vi "Status Queue.vi"(5 "All Status":bool, 7 "Action":T1=enum."Enqueue", 8 "Error In":errorcluster, 11 "Status Message [In]":string="Status Message") -> (0 "Error Out":errorcluster, 3 "Status Message [Out]":string="Status Message")   [LabVIEW 2017]
uses:
  Controls/Queue Manager Actions.ctl
  Controls/QueueNames.ctl
  Controls/MessagePacket.ctl
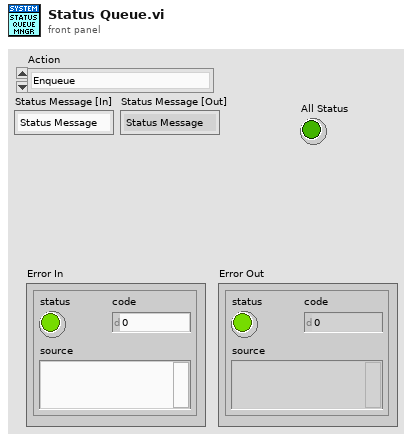
[diagram p1: front panel]
types:
  T1 = typedef "Queue Manager Actions.ctl" = enum16{"Init", "Enqueue", "Enqueue All", "Preview Queue", "Dequeue", "Get Status", "Flush Queue", "Flush All Queues", "Release All Queues", "Release Queue", "Enqueue at Opposite End"}
  T2 = typedef "MessagePacket.ctl" = cluster{"Message":string, "Parameter":variant}
  T3 = typedef "QueueNames.ctl" = enum16{"Main GUI", "Main Scan Processor", "Main Display", "Main Table Stage GUI", "Main Table Stage Proc.", "Scan Engine", "Vibratome GUI", "Vibratome Processor", "Slice Engine"}
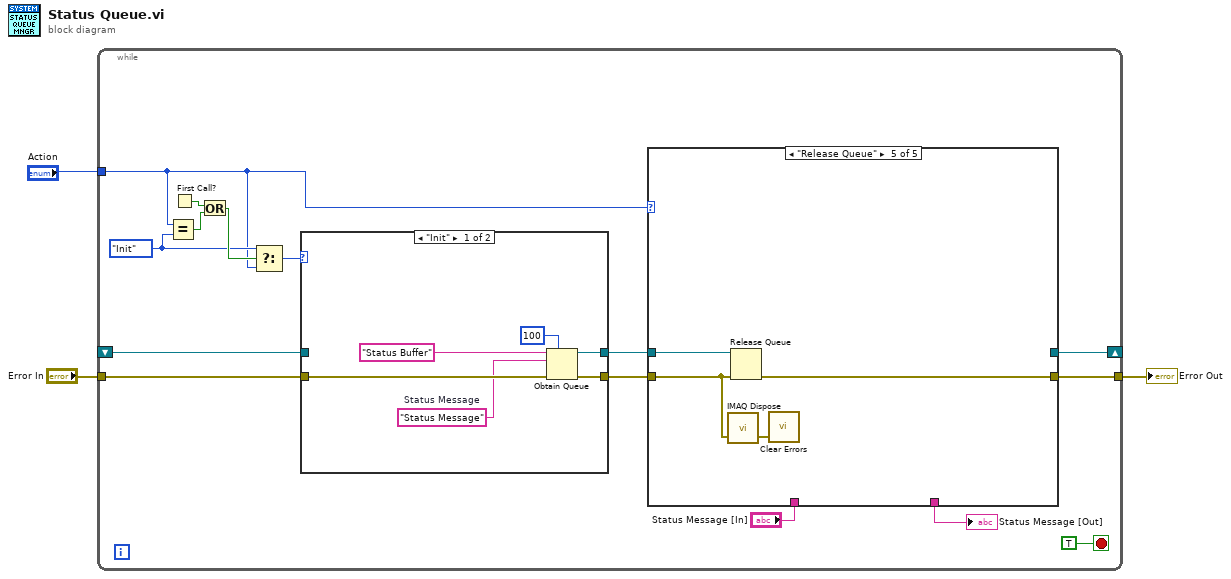
[diagram p0: block diagram]
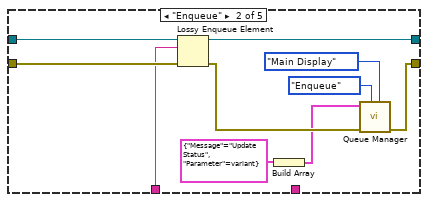
[diagram p3: hidden frame]
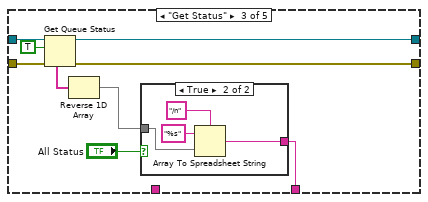
[diagram p4: hidden frame]
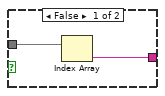
[diagram p5: hidden frame]
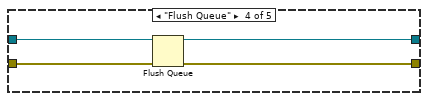
[diagram p6: hidden frame]
diagram:
  n1 = while {
    tunnel: "Action" -> [w6]
    tunnel: "Error In" -> [w13]
    tunnel: [w12] -> w1
    shift-right: [w8] -> _
    shift-left: _ -> [w7]
    stop <- TRUE stop-if-true
    w15 = Queue_Manager_Actions."Init"
    n2 = Equal?(x=w6, y=w15) -> (x = y?=w17:bool)
    n3 = First Call?() -> (First Call?: T/F=w18:bool)
    n4 = Or(x=w18, y=w17) -> (x .or. y?=w16:bool)
    n5 = Select(t=w15, s=w16, f=w6) -> (s? t:f=w14:T1)
    n6 = case shown="\"Init\"" w14 {
      tunnel: [w59 w60] -> w10
      tunnel: w13 -> [w56 w61]
      tunnel: [w58 w61] -> w11
      tunnel: w7 -> [_ w60]
      frame "Init" {
        w55 = "Status Message"  # Status Message
        n7 = Obtain Queue(max queue size (-1, unlimited)=100, name (unnamed)="Status Buffer", element data type=w55, error in (no error)=w56) -> (queue out=w59:refnum<queue>, error out=w58:errorcluster)  [unwired: 1 in, 1 out]
      }
      frame "Enqueue", Default {
      }
    }
    n8 = case shown="\"Release Queue\"" w6 {
      tunnel: w10 -> [w19 w30 w37 w47 w52]
      tunnel: [w20 w23 w38 w48 w53] -> w12
      tunnel: w11 -> [w20 w28 w39 w49 w51]
      tunnel: [w19 w29 w36 w46 _] -> w8
      tunnel: "Status Message [In]" -> [_ w27 _ _ _]
      tunnel: [_ _ w32 _ _] -> w4
      frame "Init", Default {
      }
      frame "Enqueue" {
        n9 = Lossy Enqueue Element(queue=w30, element=w27, error in (no error)=w28) -> (queue out=w29:refnum<queue>, error out=w24:errorcluster)  [unwired: 2 out]
        n10 = Build Array(T2 {"Message"="Update Status", "Parameter"=variant} ("Message Packet")) -> (w21:T2[])
        n11 = call "Queue Manager.vi"("Queue Name"=QueueNames."Main Display", "Action"=Queue_Manager_Actions."Enqueue", "Error In"=w24, "Message Packet Array"=w21) -> ("Error Out"=w23:errorcluster)  [unwired: 3 in, 4 out]
      }
      frame "Get Status" {
        n12 = Get Queue Status(queue=w37, return elements? (F)=TRUE, error in (no error)=w39) -> (queue out=w36:refnum<queue>, error out=w38:errorcluster, elements=w34:string[])  [unwired: 5 out]
        n13 = Reverse 1D Array(array=w34) -> (reversed array=w33:string[])
        n14 = case shown="True" "All Status" {
          tunnel: w33 -> [w41 w45]
          tunnel: [w40 w44] -> w32
          frame False {
            n15 = Index Array(array=w41) -> (element=w40:string)  [unwired: 1 in]
          }
          frame True {
            n16 = Array To Spreadsheet String(delimiter (Tab)="/n", array=w45, 3:"%s" ("format string")) -> (spreadsheet string=w44:string)
          }
        }
      }
      frame "Flush Queue" {
        n17 = Flush Queue(queue=w47, error in (no error)=w49) -> (queue out=w46:refnum<queue>, error out=w48:errorcluster)  [unwired: 1 out]
      }
      frame "Release Queue" {
        n18 = call "IMAQ Dispose"("error in (no error)"=w51) -> ("error out"=w50:errorcluster)  [unwired: 5 in]
        n19 = Release Queue(queue=w52, error in (no error)=w51) -> (error out=w53:errorcluster)  [unwired: 1 in, 2 out]
        n20 = call <vilib>:"Clear Errors.vi"("error in (no error)"=w50) -> ()  [unwired: 5 in, 2 out]
      }
    }
    "Status Message [Out]" <- w4
  }
  "Error Out" <- w1
